vi "Func-엑셀 데이터를 그래프로 출력.vi"() -> ()   [LabVIEW 2015] (continued)
\n1094.48\n1094.65\n1094.81\n1094.98\n1095.15\n1095.31\n1095.48\n1095.65\n1095.81\n1095.98\n1096.15\n1096.31\n1096.48\n1096.66\n1096.82\n1096.99\n1097.16\n1097.32\n1097.49\n1097.66\n1097.82\n1097.99\n1098.16\n1098.32\n1098.5\n1098.66\n1098.83\n1099\n1099.16\n1099.33\n1099.5\n1099.66\n1099.83\n1100\n1100.16\n1100.33\n1100.5\n1100.66\n1100.83\n1101\n1101.16\n1101.33\n1101.5\n1101.66\n1101.83\n1102\n1102.16\n1102.33\n1102.5\n1102.66\n1102.83\n1103\n1103.17\n1103.33\n1103.5\n1103.66\n1103.83\n1104\n1104.16\n1104.33\n1104.5\n1104.66\n1104.84\n1105.01\n1105.17\n1105.34\n1105.51\n1105.67\n1105.84\n1106.01\n1106.17\n1106.34\n1106.51\n1106.67\n1106.84\n1107.01\n1107.17\n1107.35\n1107.51\n1107.68\n1107.85\n1108.02\n1108.19\n1108.36\n1108.53\n1108.7\n1108.86\n1109.03\n1109.2\n1109.36\n1109.53\n1109.7\n1109.86\n1110.03\n1110.2\n1110.36\n1110.54\n1110.71\n1110.87\n1111.04\n1111.21\n1111.37\n1111.54\n1111.71\n1111.87\n1112.04\n1112.21\n1112.37\n1112.54\n1112.71\n1112.87\n1113.04\n1113.21\n1113.37\n1113.54\n1113.71\n1113.87\n1114.04\n1114.21\n1114.37\n1114.54\n1114.71\n1114.87\n1115.04\n1115.21\n1115.37\n1115.54\n1115.71\n1115.87\n1116.04\n1116.21\n1116.37\n1116.54\n1116.71\n1116.87\n1117.04\n1117.21\n1117.37\n1117.54\n1117.71\n1117.87\n1118.04\n1118.21\n1118.37\n1118.54\n1118.71\n1118.87\n1119.04\n1119.21\n1119.37\n1119.54\n1119.71\n1119.87\n1120.04\n1120.21\n1120.37\n1120.54\n1120.71\n1120.89\n1121.06\n1121.22\n1121.39\n1121.56\n1121.72\n1121.89\n1122.06\n1122.22\n1122.39\n1122.56\n1122.72\n1122.89\n1123.06\n1123.22\n1123.39\n1123.56\n1123.72\n1123.89\n1124.05\n1124.06\n1124.08\n1124.09\n1124.11\n1124.13\n1124.14\n1124.16\n1124.18\n1124.19\n1124.21\n1124.23\n1124.24\n1124.26\n1124.28\n1124.3\n1124.31\n1124.33\n1124.34\n1124.36\n1124.38\n1124.4\n1124.41\n1124.43\n1124.44\n1124.46\n1124.48\n1124.49\n1124.51\n1124.53\n1124.55\n1124.56\n1124.58\n1124.59\n1124.61\n1124.63\n1124.65\n1124.66\n1124.68\n1124.69\n1124.71\n1124.73\n1124.74\n1124.76\n1124.78\n1124.79\n1124.81\n1124.83\n1124.84\n1124.86\n1124.88\n1124.9\n1124.91\n1124.93\n1124.94\n1124.96\n1124.98\n1124.99\n1125.01\n1125.03\n1125.04\n1125.06\n1125.08\n1125.09\n1125.11\n1125.13\n1125.14\n1125.16\n1125.18\n1125.2\n1125.21\n1125.23\n1125.24\n1125.26\n1125.28\n1125.29\n1125.31\n1125.33\n1125.34\n1125.36\n1125.38\n1125.39\n1125.41\n1125.43\n1125.44\n1125.46\n1125.48\n1125.49\n1125.51\n1125.53\n1125.54\n1125.56\n1125.58\n1125.59\n1125.61\n1125.63\n1125.64\n1125.66\n1125.68\n1125.69\n1125.71\n1125.73\n1125.74\n1125.76\n1125.78\n1125.8\n1125.81\n1125.83\n1125.84\n1125.86\n1125.88\n1125.89\n1125.91\n1125.93\n1125.94\n1125.96\n1125.98\n1125.99\n1126.01\n1126.03\n1126.04\n1126.06\n1126.08\n1126.09\n1126.11\n1126.13\n1126.14\n1126.16\n1126.18\n1126.19\n1126.21\n1126.23\n1126.24\n1126.26\n1126.28\n1126.29\n1126.31\n1126.33\n1126.34\n1126.36\n1126.38\n1126.39\n1126.41\n1126.43\n1126.44\n1126.46\n1126.48\n1126.49\n1126.51\n1126.53\n1126.54\n1126.56\n1126.58\n1126.59\n1126.61\n1126.63\n1126.64\n1126.66\n1126.68\n1126.69\n1126.71\n1126.73\n1126.74\n1126.76\n1126.78\n1126.79\n1126.81\n1126.83\n1126.84\n1126.86\n1126.88\n1126.89\n1126.91\n1126.93\n1126.94\n1126.96\n1126.98\n1126.99\n1127.01\n1127.03\n1127.05\n1127.06\n1127.08\n1127.09\n1127.11\n1127.13\n1127.14\n1127.16\n1127.18\n1127.19\n1127.21\n1127.23\n1127.24\n1127.26\n1127.28\n1127.29\n1127.31\n1127.33\n1127.34\n1127.36\n1127.38\n1127.4\n1127.41\n1127.43\n1127.44\n1127.46\n1127.48\n1127.49\n1127.51\n1127.53\n1127.54\n1127.56\n1127.58\n1127.59\n1127.61\n1127.63\n1127.65\n1127.66\n1127.68\n1127.69\n1127.71\n1127.73\n1127.75\n1127.76\n1127.78\n1127.79\n1127.81\n1127.83\n1127.84\n1127.86\n1127.88\n1127.89\n1127.91\n1127.93\n1127.94\n1127.96\n1127.98\n1127.99\n1128.01\n1128.03\n1128.04\n1128.06\n1128.08\n1128.09\n1128.11\n1128.13\n1128.14\n1128.16\n1128.18\n1128.19\n1128.21\n1128.23\n1128.24\n1128.26\n1128.28\n1128.29\n1128.31\n1128.33\n1128.34\n1128.36\n1128.38\n1128.39\n1128.41\n1128.43\n1128.44\n1128.46\n1128.48\n1128.49\n1128.51\n1128.53\n1128.54\n1128.56\n1128.58\n1128.59\n1128.61\n1128.63\n1128.64\n1128.66\n1128.68\n1128.69\n1128.71\n1128.73\n1128.74\n1128.76\n1128.78\n1128.79\n1128.81\n1128.83\n1128.84\n1128.86\n1128.88\n1128.89\n1128.91\n1128.93\n1128.94\n1128.96\n1128.98\n1128.99\n1129.01\n1129.03\n1129.04\n1129.06\n1129.08\n1129.09\n1129.11\n1129.13\n1129.14\n1129.16\n1129.18\n1129.19\n1129.21\n1129.23\n1129.24\n1129.26\n1129.28\n1129.29\n1129.31\n1129.33\n1129.34\n1129.36\n1129.38\n1129.39\n1129.41\n1129.43\n1129.44\n1129.46\n1129.48\n1129.49\n1129.51\n1129.53\n1129.54\n1129.56\n1129.58\n1129.59\n1129.61\n1129.63\n1129.64\n1129.66\n1129.68\n1129.69\n1129.71\n1129.73\n1129.74\n1129.76\n1129.78\n1129.8\n1129.81\n1129.83\n1129.84\n1129.86\n1129.88\n1129.89\n1129.91\n1129.93\n1129.94\n1129.96\n1129.98\n1129.99\n1130.01\n1130.03\n1130.04\n1130.06\n1130.08\n1130.09\n1130.11\n1130.13\n1130.15\n1130.16\n1130.18\n1130.19\n1130.21\n1130.23\n1130.24\n1130.26\n1130.28\n1130.29\n1130.31\n1130.33\n1130.34\n1130.36\n1130.38\n1130.39\n1130.41\n1130.43\n1130.44\n1130.46\n1130.48\n1130.5\n1130.51\n1130.53\n1130.54\n1130.56\n1130.58\n1130.6\n1130.61\n1130.63\n1130.64\n1130.66\n1130.68\n1130.69\n1130.71\n1130.73\n1130.74\n1130.76\n1130.78\n1130.79\n1130.81\n1130.83\n1130.84\n1130.86\n1130.88\n1130.89\n1130.91\n1130.93\n1130.94\n1130.96\n1130.98\n1130.99\n1131.01\n1131.03\n1131.04\n1131.06\n1131.08\n1131.09\n1131.11\n1131.13\n1131.14\n1131.16\n1131.18\n1131.2\n1131.21\n1131.23\n1131.24\n1131.26\n1131.28\n1131.29\n1131.31\n1131.33\n1131.34\n1131.36\n1131.38\n1131.39\n1131.41\n1131.43\n1131.44\n1131.46\n1131.48\n1131.49\n1131.51\n1131.53\n1131.54\n1131.56\n1131.58\n1131.59\n1131.61\n1131.63\n1131.64\n1131.66\n1131.68\n1131.69\n1131.71\n1131.73\n1131.74\n1131.76\n1131.78\n1131.79\n1131.81\n1131.83\n1131.84\n1131.86\n1131.88\n1131.89\n1131.91\n1131.93\n1131.94\n1131.96\n1131.98\n1131.99\n1132.01\n1132.03\n1132.04\n1132.06\n1132.08\n1132.09\n1132.11\n1132.13\n1132.14\n1132.16\n1132.18\n1132.19\n1132.21\n1132.23\n1132.24\n1132.26\n1132.28\n1132.29\n1132.31\n1132.33\n1132.34\n1132.36\n1132.38\n1132.39\n1132.41\n1132.43\n1132.44\n1132.46\n1132.48\n1132.49\n1132.51\n1132.53\n1132.54\n1132.56\n1132.58\n1132.59\n1132.61\n1132.63\n1132.64\n1132.66\n1132.68\n1132.69\n1132.71\n1132.73\n1132.74\n1132.76\n1132.78\n1132.79\n1132.81\n1132.83\n1132.84\n1132.86\n1132.88\n1132.89\n1132.91\n1132.93\n1132.94\n1132.96\n1132.98\n1132.99\n1133.01\n1133.03\n1133.04\n1133.06\n1133.08\n1133.09\n1133.11\n1133.13\n1133.14\n1133.16\n1133.18\n1133.19\n1133.21\n1133.23\n1133.25\n1133.26\n1133.28\n1133.29\n1133.31\n1133.33\n1133.34\n1133.36\n1133.38\n1133.39\n1133.41\n1133.43\n1133.44\n1133.46\n1133.48\n1133.5\n1133.51\n1133.53\n1133.54\n1133.56\n1133.58\n1133.6\n1133.61\n1133.63\n1133.64\n1133.66\n1133.68\n1133.69\n1133.71\n1133.73\n1133.75\n1133.76\n1133.78\n1133.79\n1133.81\n1133.83\n1133.85\n1133.86\n1133.88\n1133.89\n1133.91\n1133.93\n1133.94\n1133.96\n1133.98\n1133.99\n1134.01\n1134.03\n1134.04\n1134.06\n1134.08\n1134.09\n1134.11\n1134.13\n1134.14\n1134.16\n1134.18\n1134.19\n1134.21\n1134.23\n1134.24\n1134.26\n1134.28\n1134.29\n1134.31\n1134.33\n1134.34\n1134.36\n1134.38\n1134.39\n1134.41\n1134.43\n1134.44\n1134.46\n1134.48\n1134.49\n1134.51\n1134.53\n1134.54\n1134.56\n1134.58\n1134.59\n1134.61\n1134.63\n1134.64\n1134.66\n1134.68\n1134.69\n1134.71\n1134.73\n1134.74\n1134.76\n1134.78\n1134.79\n1134.81\n1134.83\n1134.84\n1134.86\n1134.88\n1134.89\n1134.91\n1134.93\n1134.94\n1134.96\n1134.98\n1134.99\n1135.01\n1135.03\n1135.04\n1135.06\n1135.08\n1135.09\n1135.11\n1135.13\n1135.14\n1135.16\n1135.18\n1135.19\n1135.21\n1135.23\n1135.24\n1135.26\n1135.28\n1135.29\n1135.31\n1135.33\n1135.34\n1135.36\n1135.38\n1135.39\n1135.41\n1135.43\n1135.44\n1135.46\n1135.48\n1135.49\n1135.51\n1135.53\n1135.54\n1135.56\n1135.58\n1135.59\n1135.61\n1135.63\n1135.64\n1135.66\n1135.68\n1135.69\n1135.71\n1135.73\n1135.74\n1135.76\n1135.78\n1135.79\n1135.81\n1135.83\n1135.84\n1135.86\n1135.88\n1135.89\n1135.91\n1135.93\n1135.94\n1135.96\n1135.98\n1135.99\n1136.01\n1136.03\n1136.04\n1136.06\n1136.08\n1136.09\n1136.11\n1136.13\n1136.14\n1136.16\n1136.18\n1136.19\n1136.21\n1136.23\n1136.24\n1136.26\n1136.28\n1136.29\n1136.31\n1136.33\n1136.35\n1136.36\n1136.38\n1136.39\n1136.41\n1136.43\n1136.44\n1136.46\n1136.48\n1136.49\n1136.51\n1136.53\n1136.54\n1136.56\n1136.58\n1136.6\n1136.61\n1136.63\n1136.64\n1136.66\n1136.68\n1136.7\n1136.71\n1136.73\n1136.74\n1136.76\n1136.78\n1136.79\n1136.81\n1136.83\n1136.84\n1136.86\n1136.88\n1136.89\n1136.91\n1136.93\n1136.95\n1136.96\n1136.98\n1136.99\n1137.01\n1137.03\n1137.04\n1137.06\n1137.08\n1137.09\n1137.11\n1137.13\n1137.14\n1137.16\n1137.18\n1137.2\n1137.21\n1137.23\n1137.24\n1137.26\n1137.28\n1137.3\n1137.31\n1137.33\n1137.34\n1137.36\n1137.38\n1137.39\n1137.41\n1137.43\n1137.44\n1137.46\n1137.48\n1137.49\n1137.51\n1137.53\n1137.54\n1137.56\n1137.58\n1137.59\n1137.61\n1137.63\n1137.65\n1137.66\n1137.68\n1137.69\n1137.71\n1137.73\n1137.74\n1137.76\n1137.78\n1137.79\n1137.81\n1137.83\n1137.84\n1137.86\n1137.88\n1137.89\n1137.91\n1137.93\n1137.94\n1137.96\n1137.98\n1137.99\n1138.01\n1138.03\n1138.04\n1138.06\n1138.08\n1138.09\n1138.11\n1138.13\n1138.14\n1138.16\n1138.18\n1138.19\n1138.21\n1138.23\n1138.24\n1138.26\n1138.28\n1138.29\n1138.31\n1138.33\n1138.34\n1138.36\n1138.38\n1138.39\n1138.41\n1138.43\n1138.44\n1138.46\n1138.48\n1138.49\n1138.51\n1138.53\n1138.54\n1138.56\n1138.58\n1138.59\n1138.61\n1138.63\n1138.64\n1138.66\n1138.68\n1138.69\n1138.71\n1138.73\n1138.74\n1138.76\n1138.78\n1138.79\n1138.81\n1138.83\n1138.84\n1138.86\n1138.88\n1138.89\n1138.91\n1138.93\n1138.94\n1138.96\n1138.98\n1138.99\n1139.01\n1139.03\n1139.04\n1139.06\n1139.08\n1139.09\n1139.11\n1139.13\n1139.14\n1139.16\n1139.18\n1139.19\n1139.21\n1139.23\n1139.24\n1139.26\n1139.28\n1139.29\n1139.31\n1139.33\n1139.35\n1139.36\n1139.38\n1139.39\n1139.41\n1139.43\n1139.45\n1139.46\n1139.48\n1139.49\n1139.51\n1139.53\n1139.54\n1139.56\n1139.58\n1139.59\n1139.61\n1139.63\n1139.64\n1139.66\n1139.68\n1139.7\n1139.71\n1139.73\n1139.74\n1139.76\n1139.78\n1139.8\n1139.81\n1139.83\n1139.84\n1139.86\n1139.88\n1139.89\n1139.91\n1139.93\n1139.95\n1139.96\n1139.98\n1139.99\n1140.01\n1140.03\n1140.05\n1140.06\n1140.08\n1140.09\n1140.11\n1140.13\n1140.15\n1140.16\n1140.18\n1140.19\n1140.21\n1140.23\n1140.24\n1140.26\n1140.28\n1140.3\n1140.31\n1140.33\n1140.34\n1140.36\n1140.38\n1140.39\n1140.41\n1140.43\n1140.44\n1140.46\n1140.48\n1140.49\n1140.51\n1140.53\n1140.54\n1140.56\n1140.58\n1140.6\n1140.61\n1140.63\n1140.64\n1140.66\n1140.68\n1140.69\n1140.71\n1140.73\n1140.75\n1140.76\n1140.78\n1140.79\n1140.81\n1140.83\n1140.85\n1140.86\n1140.88\n1140.89\n1140.91\n1140.93\n1140.94\n1140.96\n1140.98\n1140.99\n1141.01\n1141.03\n1141.04\n1141.06\n1141.08\n1141.09\n1141.11\n1141.13\n1141.14\n1141.16\n1141.18\n1141.19\n1141.21\n1141.23\n1141.24\n1141.26\n1141.28\n1141.29\n1141.31\n1141.33\n1141.34\n1141.36\n1141.38\n1141.39\n1141.41\n1141.43\n1141.44\n1141.46\n1141.48\n1141.49\n1141.51\n1141.53\n1141.54\n1141.56\n1141.58\n1141.59\n1141.61\n1141.63\n1141.64\n1141.66\n1141.68\n1141.69\n1141.71\n1141.73\n1141.74\n1141.76\n1141.78\n1141.79\n1141.81\n1141.83\n1141.84\n1141.86\n1141.88\n1141.89\n1141.91\n1141.93\n1141.94\n1141.96\n1141.98\n1141.99\n1142.01\n1142.03\n1142.04\n1142.06\n1142.08\n1142.09\n1142.11\n1142.13\n1142.14\n1142.16\n1142.18\n1142.19\n1142.21\n1142.23\n1142.24\n1142.26\n1142.28\n1142.29\n1142.31\n1142.33\n1142.34\n1142.36\n1142.38\n1142.39\n1142.41\n1142.43\n1142.44\n1142.46\n1142.48\n1142.49\n1142.51\n1142.53\n1142.55\n1142.56\n1142.58\n1142.59\n1142.61\n1142.63\n1142.64\n1142.66\n1142.68\n1142.69\n1142.71\n1142.73\n1142.74\n1142.76\n1142.78\n1142.8\n1142.81\n1142.83\n1142.84\n1142.86\n1142.88\n1142.9\n1142.91\n1142.93\n1142.94\n1142.96\n1142.98\n1142.99\n1143.01\n1143.03\n1143.05\n1143.06\n1143.08\n1143.09\n1143.11\n1143.13\n1143.15\n1143.16\n1143.18\n1143.19\n1143.21\n1143.23\n1143.25\n1143.26\n1143.28\n1143.29\n1143.31\n1143.33\n1143.34\n1143.36\n1143.38\n1143.39\n1143.41\n1143.43\n1143.44\n1143.46\n1143.48\n1143.49\n1143.51\n1143.53\n1143.54\n1143.56\n1143.58\n1143.59\n1143.61\n1143.63\n1143.64\n1143.66\n1143.68\n1143.69\n1143.71\n1143.73\n1143.74\n1143.76\n1143.78\n1143.79\n1143.81\n1143.83\n1143.84\n1143.86\n1143.88\n1143.89\n1143.91\n1143.93\n1143.94\n1143.96\n1143.98\n1143.99\n1144.01\n1144.03\n1144.04\n1144.06\n1144.08\n1144.09\n1144.11\n1144.13\n1144.14\n1144.16\n1144.18\n1144.19\n1144.21\n1144.23\n1144.24\n1144.26\n1144.28\n1144.29\n1144.31\n1144.33\n1144.34\n1144.36\n1144.38\n1144.39\n1144.41\n1144.43\n1144.44\n1144.46\n1144.48\n1144.49\n1144.51\n1144.53\n1144.54\n1144.56\n1144.58\n1144.59\n1144.61\n1144.63\n1144.64\n1144.66\n1144.68\n1144.69\n1144.71\n1144.73\n1144.74\n1144.76\n1144.78\n1144.79\n1144.81\n1144.83\n1144.84\n1144.86\n1144.88\n1144.89\n1144.91\n1144.93\n1144.94\n1144.96\n1144.98\n1144.99\n1145.01\n1145.03\n1145.04\n1145.06\n1145.08\n1145.09\n1145.11\n1145.13\n1145.14\n1145.16\n1145.18\n1145.2\n1145.21\n1145.23\n1145.24\n1145.26\n1145.28\n1145.29\n1145.31\n1145.33\n1145.34\n1145.36\n1145.38\n1145.39\n1145.41\n1145.43\n1145.44\n1145.46\n1145.48\n1145.49\n1145.51\n1145.53\n1145.54\n1145.56\n1145.58\n1145.59\n1145.61\n1145.63\n1145.64\n1145.66\n1145.68\n1145.69\n1145.71\n1145.73\n1145.74\n1145.76\n1145.78\n1145.79\n1145.81\n1145.83\n1145.84\n1145.86\n1145.88\n1145.9\n1145.91\n1145.93\n1145.94\n1145.96\n1145.98\n1145.99\n1146.01\n1146.03\n1146.04\n1146.06\n1146.08\n1146.09\n1146.11\n1146.13\n1146.14\n1146.16\n1146.18\n1146.19\n1146.21\n1146.23\n1146.25\n1146.26\n1146.28\n1146.29\n1146.31\n1146.33\n1146.35\n1146.36\n1146.38\n1146.39\n1146.41\n1146.43\n1146.44\n1146.46\n1146.48\n1146.5\n1146.51\n1146.53\n1146.54\n1146.56\n1146.58\n1146.59\n1146.61\n1146.63\n1146.64\n1146.66\n1146.68\n1146.7\n1146.71\n1146.73\n1146.74\n1146.76\n1146.78\n1146.79\n1146.81\n1146.83\n1146.84\n1146.86\n1146.88\n1146.89\n1146.91\n1146.93\n1146.95\n1146.96\n1146.98\n1146.99\n1147.01\n1147.03\n1147.05\n1147.06\n1147.08\n1147.09\n1147.11\n1147.13\n1147.14\n1147.16\n1147.18\n1147.19\n1147.21\n1147.23\n1147.24\n1147.26\n1147.28\n1147.29\n1147.31\n1147.33\n1147.34\n1147.36\n1147.38\n1147.39\n1147.41\n1147.43\n1147.44\n1147.46\n1147.48\n1147.49\n1147.51\n1147.53\n1147.54\n1147.56\n1147.58\n1147.59\n1147.61\n1147.63\n1147.64\n1147.66\n1147.68\n1147.69\n1147.71\n1147.73\n1147.74\n1147.76\n1147.78\n1147.79\n1147.81\n1147.83\n1147.84\n1147.86\n1147.88\n1147.89\n1147.91\n1147.93\n1147.94\n1147.96\n1147.98\n1147.99\n1148.01\n1148.03\n1148.04\n1148.06\n1148.08\n1148.09\n1148.11\n1148.13\n1148.14\n1148.16\n1148.18\n1148.19\n1148.21\n1148.23\n1148.24\n1148.26\n1148.28\n1148.29\n1148.31\n1148.33\n1148.34\n1148.36\n1148.38\n1148.39\n1148.41\n1148.43\n1148.44\n1148.46\n1148.48\n1148.49\n1148.51\n1148.53\n1148.54\n1148.56\n1148.58\n1148.59\n1148.61\n1148.63\n1148.64\n1148.66\n1148.68\n1148.69\n1148.71\n1148.73\n1148.74\n1148.76\n1148.78\n1148.79\n1148.81\n1148.83\n1148.84\n1148.86\n1148.88\n1148.89\n1148.91\n1148.93\n1148.94\n1148.96\n1148.98\n1149\n1149.01\n1149.03\n1149.04\n1149.06\n1149.08\n1149.09\n1149.11\n1149.13\n1149.14\n1149.16\n1149.18\n1149.19\n1149.21\n1149.23\n1149.25\n1149.26\n1149.28\n1149.29\n1149.31\n1149.33\n1149.35\n1149.36\n1149.38\n1149.39\n1149.41\n1149.43\n1149.44\n1149.46\n1149.48\n1149.49\n1149.51\n1149.53\n1149.54\n1149.56\n1149.58\n1149.6\n1149.61\n1149.63\n1149.64\n1149.66\n1149.68\n1149.69\n1149.71\n1149.73\n1149.74\n1149.76\n1149.78\n1149.8\n1149.81\n1149.83\n1149.84\n1149.86\n1149.88\n1149.89\n1149.91\n1149.93\n1149.94\n1149.96\n1149.98\n1149.99\n1150.01\n1150.03\n1150.05\n1150.06\n1150.08\n1150.09\n1150.11\n1150.13\n1150.15\n1150.16\n1150.18\n1150.19\n1150.21\n1150.23\n1150.24\n1150.26\n1150.28\n1150.3\n1150.31\n1150.33\n1150.34\n1150.36\n1150.38\n1150.39\n1150.41\n1150.43\n1150.44\n1150.46\n1150.48\n1150.49\n1150.51\n1150.53\n1150.54\n1150.56\n1150.58\n1150.59\n1150.61\n1150.63\n1150.64\n1150.66\n1150.68\n1150.69\n1150.71\n1150.73\n1150.74\n1150.76\n1150.78\n1150.79\n1150.81\n1150.83\n1150.84\n1150.86\n1150.88\n1150.89\n1150.91\n1150.93\n1150.94\n1150.96\n1150.98\n1150.99\n1151.01\n1151.03\n1151.04\n1151.06\n1151.08\n1151.09\n1151.11\n1151.13\n1151.14\n1151.16\n1151.18\n1151.19\n1151.21\n1151.23\n1151.24\n1151.26\n1151.28\n1151.29\n1151.31\n1151.33\n1151.34\n1151.36\n1151.38\n1151.39\n1151.41\n1151.43\n1151.44\n1151.46\n1151.48\n1151.49\n1151.51\n1151.53\n1151.54\n1151.56\n1151.58\n1151.59\n1151.61\n1151.63\n1151.64\n1151.66\n1151.68\n1151.69\n1151.71\n1151.73\n1151.75\n1151.76\n1151.78\n1151.79\n1151.81\n1151.83\n1151.84\n1151.86\n1151.88\n1151.89\n1151.91\n1151.93\n1151.94\n1151.96\n1151.98\n1151.99\n1152.01\n1152.03\n1152.04\n1152.06\n1152.08\n1152.1\n1152.11\n1152.13\n1152.14\n1152.16\n1152.18\n1152.19\n1152.21\n1152.23\n1152.24\n1152.26\n1152.28\n1152.29\n1152.31\n1152.33\n1152.35\n1152.36\n1152.38\n1152.39\n1152.41\n1152.43\n1152.45\n1152.46\n1152.48\n1152.49\n1152.51\n1152.53\n1152.55\n1152.56\n1152.58\n1152.59\n1152.61\n1152.63\n1152.64\n1152.66\n1152.68\n1152.69\n1152.71\n1152.73\n1152.74\n1152.76\n1152.78\n1152.79\n1152.81\n1152.83\n1152.84\n1152.86\n1152.88\n1152.89\n1152.91\n1152.93\n1152.95\n1152.96\n1152.98\n1152.99\n1153.01\n1153.03\n1153.05\n1153.06\n1153.08\n1153.09\n1153.11\n1153.13\n1153.14\n1153.16\n1153.18\n1153.19\n1153.21\n1153.23\n1153.24\n1153.26\n1153.28\n1153.29\n1153.31\n1153.33\n1153.34\n1153.36\n1153.38\n1153.39\n1153.41\n1153.43\n1153.44\n1153.46\n1153.48\n1153.49\n1153.51\n1153.53\n1153.54\n1153.56\n1153.58\n1153.59\n1153.61\n1153.63\n1153.64\n1153.66\n1153.68\n1153.69\n1153.71\n1153.73\n1153.75\n1153.76\n1153.78\n1153.79\n1153.81\n1153.83\n1153.84\n1153.86\n1153.88\n1153.89\n1153.91\n1153.93\n1153.94\n1153.96\n1153.98\n1153.99\n1154.01\n1154.03\n1154.04\n1154.06\n1154.08\n1154.09\n1154.11\n1154.13\n1154.14\n1154.16\n1154.18\n1154.19\n1154.21\n1154.23\n1154.24\n1154.26\n1154.28\n1154.29\n1154.31\n1154.33\n1154.34\n1154.36\n1154.38\n1154.39\n1154.41\n1154.43\n1154.44\n1154.46\n1154.48\n1154.49\n1154.51\n1154.53\n1154.54\n1154.56\n1154.58\n1154.59\n1154.61\n1154.63\n1154.64\n1154.66\n1154.68\n1154.69\n1154.71\n1154.73\n1154.74\n1154.76\n1154.78\n1154.79\n1154.81\n1154.83\n1154.85\n1154.86\n1154.88\n1154.89\n1154.91\n1154.93\n1154.94\n1154.96\n1154.98\n1154.99\n1155.01\n1155.03\n1155.04\n1155.06\n1155.08\n1155.1\n1155.11\n1155.13\n1155.14\n1155.16\n1155.18\n1155.2\n1155.21\n1155.23\n1155.24\n1155.26\n1155.28\n1155.29\n1155.31\n1155.33\n1155.34\n1155.36\n1155.38\n1155.39\n1155.41\n1155.43\n1155.45\n1155.46\n1155.48\n1155.49\n1155.51\n1155.53\n1155.55\n1155.56\n1155.58\n1155.59\n1155.61\n1155.63\n1155.64\n1155.66\n1155.68\n1155.69\n1155.71\n1155.73\n1155.74\n1155.76\n1155.78\n1155.8\n1155.81\n1155.83\n1155.84\n1155.86\n1155.88\n1155.9\n1155.91\n1155.93\n1155.94\n1155.96\n1155.98\n1156\n1156.01\n1156.03\n1156.04\n1156.06\n1156.08\n1156.09\n1156.11\n1156.13\n1156.14\n1156.16\n1156.18\n1156.19\n1156.21\n1156.23\n1156.24\n1156.26\n1156.28\n1156.29\n1156.31\n1156.33\n1156.34\n1156.36\n1156.38\n1156.39\n1156.41\n1156.43\n1156.44\n1156.46\n1156.48\n1156.49\n1156.51\n1156.53\n1156.54\n1156.56\n1156.58\n1156.59\n1156.61\n1156.63\n1156.64\n1156.66\n1156.68\n1156.69\n1156.71\n1156.73\n1156.74\n1156.76\n1156.78\n1156.79\n1156.81\n1156.83\n1156.84\n1156.86\n1156.88\n1156.89\n1156.91\n1156.93\n1156.94\n1156.96\n1156.98\n1156.99\n1157.01\n1157.03\n1157.04\n1157.06\n1157.08\n1157.09\n1157.11\n1157.13\n1157.14\n1157.16\n1157.18\n1157.19\n1157.21\n1157.23\n1157.24\n1157.26\n1157.28\n1157.29\n1157.31\n1157.33\n1157.34\n1157.36\n1157.38\n1157.39\n1157.41\n1157.43\n1157.44\n1157.46\n1157.48\n1157.49\n1157.51\n1157.53\n1157.54\n1157.56\n1157.58\n1157.59\n1157.61\n1157.63\n1157.64\n1157.66\n1157.68\n1157.69\n1157.71\n1157.73\n1157.74\n1157.76\n1157.78\n1157.79\n1157.81\n1157.83\n1157.85\n1157.86\n1157.88\n1157.89\n1157.91\n1157.93\n1157.94\n1157.96\n1157.98\n1157.99\n1158.01\n1158.03\n1158.04\n1158.06\n1158.08\n1158.09\n1158.11\n1158.13\n1158.14\n1158.16\n1158.18\n1158.2\n1158.21\n1158.23\n1158.24
